vi "PMA Daten speichern.vi"(6 "Aktion":T2, 8 "error in (no error)":errorcluster caption="Fehler (Eingang, kein Fehler)", 11 "PMA Daten allgemein":T1) -> (0 "error out":errorcluster caption="Fehler (Ausgang)", 3 "PMA Daten allgemein":T1)   [LabVIEW 2020, in "ABB-EL3000.lvlib" / "PMA.lvlib"]
uses:
  PMA.lvlib
  Aktion PMA Daten allgemein.ctl
  PMA Daten allgemein.ctl
  Allgemein/allgemeine Sub-VIs.lvlib
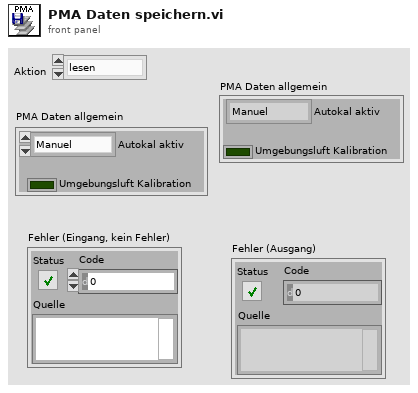
[diagram p1: front panel]
types:
  T1 = typedef "ABB-EL3000.lvlib/PMA.lvlib/PMA Daten allgemein.ctl" = cluster{"Autokal aktiv":enum16{"Manuel", "Automatic"}, "Umgebungsluft Kalibration":bool}
  T2 = typedef "ABB-EL3000.lvlib/PMA.lvlib/Aktion PMA Daten allgemein.ctl" = enum16{"lesen", "schreiben", "laden ", "speichern"}
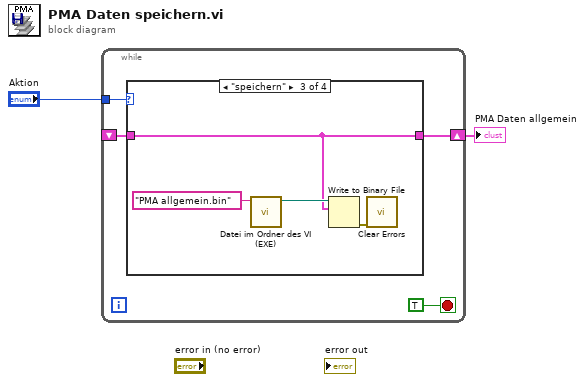
[diagram p0: block diagram]
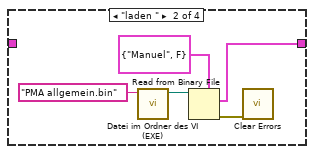
[diagram p3: hidden frame]
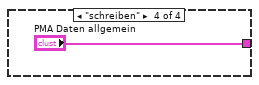
[diagram p4: hidden frame]
diagram:
  n1 = while {
    tunnel: "Aktion" -> [w5]
    shift-right: [w4] -> w1
    shift-left: _ -> [w3]
    stop <- TRUE stop-if-true
    n2 = case shown="\"speichern\"" w5 {
      tunnel: [w7 w10 w15 "PMA Daten allgemein"] -> w4
      tunnel: w3 -> [w7 _ w15 _]
      frame "lesen", Default {
      }
      frame "laden " {
        n3 = call "Datei im Ordner des VI (EXE).vi"("Dateiname"="PMA allgemein.bin") -> ("Dateipfad im Ordner des Haupt-VIs"=w11:path)  [unwired: 8 in, 2 out]
        n4 = Read from Binary File(5:T1 {"Autokal aktiv"=enum."Manuel", "Umgebungsluft Kalibration"=FALSE} ("PMA Daten allgemein"), 11:w11) -> (0:w8:errorcluster, 2:w10:T1)  [unwired: 1 in, 5 out]
        n5 = call <vilib>:"Clear Errors.vi"("error in (no error)"=w8) -> ()  [unwired: 5 in, 2 out]
      }
      frame "speichern" {
        n6 = call "Datei im Ordner des VI (EXE).vi"("Dateiname"="PMA allgemein.bin") -> ("Dateipfad im Ordner des Haupt-VIs"=w16:path)  [unwired: 8 in, 2 out]
        n7 = Write to Binary File(file (use dialog)=w16, data=w15) -> (error out=w14:errorcluster)  [unwired: 1 in, 5 out]
        n8 = call <vilib>:"Clear Errors.vi"("error in (no error)"=w14) -> ()  [unwired: 5 in, 2 out]
      }
      frame "schreiben" {
      }
    }
  }
  "PMA Daten allgemein" <- w1
